vi "MeasLeakRate.vi"() -> ()   [LabVIEW 2011]
uses:
  <vilib>/Analysis/NI_AALPro.lvlib
panel:
  out "Pfit array":dbl[](array[numeric])=[-0.7941019304586632, -1.11]
  out "tFit array":dbl[](array[numeric])=[-20.0, 0.0]
  in  "tFit":dbl=10.0
  out "leak rate":dbl=-0.015794903477066843
  out "Polynomial Coefficients":dbl[](array[numeric])=[0.21180227710532212, -0.015794903477066843]
  out "Best Polynomial Fit":dbl[](array[numeric])=[0.21180227710532212, 0.22319040251225147, 0.23459432282271855, 0.24599824313318563, 0.257386368540115, 0.2688060837540049, 0.28019420916104915, 0.29158233456797844, 0.3029704599749078, 0.31435858538195205, 0.3257467107888814, 0.3371190412923879, 0.34849137179589446, 0.35987949720282375, 0.37128341751329086, 0.3826715429202202, 0.3940754632306873, 0.4054635886376166, 0.41685171404454596, 0.428255634355013, 0.43962796485851957, 0.45100029536202607, 0.4623884207689554, 0.47377654617588477, 0.48516467158292903, 0.49653700208643553, 0.5079409223967877, 0.5193132529002942, 0.5306855834038007, 0.5420737088107301, 0.5534776291211971, 0.5648657545282414, 0.5762538799351707, 0.5876735951490606, 0.59906172055599, 0.610465640866457, 0.6218379713699635, 0.6332260967768929, 0.6446142221839373, 0.6559865526873288, 0.667374678094373, 0.6787470085978795, 0.6901509289082317, 0.701539054315276, 0.7129271797222052, 0.7242837153221742, 0.7356718407292184, 0.7470757610396854, 0.7584480915430771, 0.7698520118535441, 0.7812401372604734, 0.7926124677639799, 0.8040005931710241, 0.8153729236744158, 0.8267610490814601, 0.8381333795849666, 0.8495215049918958, 0.8609096303988253, 0.8723135507092923, 0.8837016761162217]
  out "weight array":dbl[](array[numeric])=[1.0, 0.9304378473743352, 0.8656280206959002, 0.8053325349226013, 0.7493118702139018, 0.6970486998519578, 0.6485604918048629, 0.6034452278869568, 0.5614682788434552, 0.5224113367356974, 0.48607127959631125, 0.4523043432308019, 0.42088316568580814, 0.391605626676799, 0.3643282616568307, 0.3389848035136151, 0.3153727520215804, 0.2934347445114793, 0.2730227920280988, 0.254005337094879, 0.2363598138676975, 0.2199401093320528, 0.20464060187819116, 0.19040536109693249, 0.17716035430743396, 0.16485318319590794, 0.15337030310847227, 0.14271580554234622, 0.13280146637772186, 0.12356351050464263, 0.1149566704860605, 0.10696003702829307, 0.0995196666076842, 0.09257834684880129, 0.08613839775547324, 0.08013841114202638, 0.07457126750886783, 0.0693839296169267, 0.06455743411509868, 0.06007268699843237, 0.05589390157677298, 0.05201100230461187, 0.04838816596555581, 0.045022180979351074, 0.041890341154525154, 0.038984154900943556, 0.03627233316771518, 0.0337457768453816, 0.031401487957797174, 0.0292142112925875, 0.02718200786781411, 0.02529369813118136, 0.023534214041295513, 0.02189931327407275, 0.020375949901689627, 0.01896045091502129, 0.017641521134619163, 0.01641433894890389, 0.015270995021825278, 0.014208711735371296]
  out "dtArray":dbl[](array[numeric])=[0.0, -0.7209999999977299, -1.4429999999993015, -2.165000000000873, -2.885999999998603, -3.6089999999967404, -4.330000000001746, -5.050999999999476, -5.771999999997206, -6.493000000002212, -7.213999999999942, -7.934000000001106, -8.65400000000227, -9.375, -10.097000000001572, -10.817999999999302, -11.540000000000873, -12.260999999998603, -12.981999999996333, -13.703999999997905, -14.423999999999069, -15.144000000000233, -15.864999999997963, -16.585999999995693, -17.3070000000007, -18.027000000001863, -18.74899999999616, -19.468999999997322, -20.188999999998487, -20.909999999996217, -21.631999999997788, -22.353000000002794, -23.074000000000524, -23.79699999999866, -24.51799999999639, -25.239999999997963, -25.959999999999127, -26.680999999996857, -27.402000000001863, -28.12199999999575, -28.843000000000757, -29.56300000000192, -30.284999999996217, -31.006000000001222, -31.726999999998952, -32.445999999996275, -33.16700000000128, -33.88900000000285, -34.60899999999674, -35.33099999999831, -36.05199999999604, -36.771999999997206, -37.49300000000221, -38.2129999999961, -38.934000000001106, -39.65400000000227, -40.375, -41.09599999999773, -41.8179999999993, -42.53899999999703]
  out "t_array":dbl[](array[numeric])=[54993.193, 54992.472, 54991.75, 54991.028, 54990.307, 54989.584, 54988.863, 54988.142, 54987.421, 54986.7, 54985.979, 54985.259, 54984.539, 54983.818, 54983.096, 54982.375, 54981.653, 54980.932, 54980.211, 54979.489, 54978.769, 54978.049, 54977.328, 54976.607, 54975.886, 54975.166, 54974.444, 54973.724, 54973.004, 54972.283, 54971.561, 54970.84, 54970.119, 54969.396, 54968.675, 54967.953, 54967.233, 54966.512, 54965.791, 54965.071, 54964.35, 54963.63, 54962.908, 54962.187, 54961.466, 54960.747, 54960.026, 54959.304, 54958.584, 54957.862, 54957.141, 54956.421, 54955.7, 54954.98, 54954.259, 54953.539, 54952.818, 54952.097, 54951.375, 54950.654]
  out "P_array":dbl[](array[numeric])=[-1.11, -1.1, -1.1, -1.1, -1.1, -1.12, -1.11, -1.1, -0.99, -0.82, -0.36, 4.91, 7.07, 8.7, 7.720000000000001, 6.69, 4.43, 3.14, 1.85, 0.05, -0.49, -0.74, -1.12, -1.12, -1.12, -1.12, -1.12, -1.12, -1.12, -1.12, -1.12, -1.12, -1.12, -1.12, -1.12, -1.12, -1.12, -1.13, -1.13, -1.13, -1.12, -1.12, -1.13, -1.13, -1.13, -1.12, -1.12, -1.13, -1.12, -1.12, -1.12, -1.12, -1.14, -1.14, -1.14, -1.12, -1.12, -1.12, -1.13, -1.13]
  out "angle (°)":dbl
  out "Status":string
  out "error out":errorcluster
  out "T-T0,P":cluster{"element":dbl, "element":dbl}[](array[cluster])
  out "XY Graph":cluster{"Value":dbl[], "Value":dbl[]}[](graph)=[{"Value"=[0.0, -0.7209999999977299, -1.4429999999993015, -2.165000000000873, -2.885999999998603, -3.6089999999967404, -4.330000000001746, -5.050999999999476, -5.771999999997206, -6.493000000002212, -7.213999999999942, -7.934000000001106, -8.65400000000227, -9.375, -10.097000000001572, -10.817999999999302, -11.540000000000873, -12.260999999998603, -12.981999999996333, -13.703999999997905, -14.423999999999069, -15.144000000000233, -15.864999999997963, -16.585999999995693, -17.3070000000007, -18.027000000001863, -18.74899999999616, -19.468999999997322, -20.188999999998487, -20.909999999996217, -21.631999999997788, -22.353000000002794, -23.074000000000524, -23.79699999999866, -24.51799999999639, -25.239999999997963, -25.959999999999127, -26.680999999996857, -27.402000000001863, -28.12199999999575, -28.843000000000757, -29.56300000000192, -30.284999999996217, -31.006000000001222, -31.726999999998952, -32.445999999996275, -33.16700000000128, -33.88900000000285, -34.60899999999674, -35.33099999999831, -36.05199999999604, -36.771999999997206, -37.49300000000221, -38.2129999999961, -38.934000000001106, -39.65400000000227, -40.375, -41.09599999999773, -41.8179999999993, -42.53899999999703], "Value"=[-1.11, -1.1, -1.1, -1.1, -1.1, -1.12, -1.11, -1.1, -0.99, -0.82, -0.36, 4.91, 7.07, 8.7, 7.720000000000001, 6.69, 4.43, 3.14, 1.85, 0.05, -0.49, -0.74, -1.12, -1.12, -1.12, -1.12, -1.12, -1.12, -1.12, -1.12, -1.12, -1.12, -1.12, -1.12, -1.12, -1.12, -1.12, -1.13, -1.13, -1.13, -1.12, -1.12, -1.13, -1.13, -1.13, -1.12, -1.12, -1.13, -1.12, -1.12, -1.12, -1.12, -1.14, -1.14, -1.14, -1.12, -1.12, -1.12, -1.13, -1.13]}, {"Value"=[-20.0, 0.0], "Value"=[-0.7941019304586632, -1.11]}]
  out "T,P":cluster{"element":dbl, "element":dbl}[](array[cluster])
  in  "Control Valve Local":bool
  in  "Exhaust Close":bool
  in  "Exhaust Open":bool
  in  "Control Close":bool
  in  "Control Open":bool
  in  "reset":bool
  in  "# points to watch":i32=60
  out "leak rate (torr/min)":string="-0.948"
  out "P":dbl=-1.11
  out "first":bool
  in  "interval (s)":dbl=0.5
  in  "stop":bool
  out "P(torr)":string=" -1.11"
  # "Pressure control valve:"
  # "Exahaust valve:"
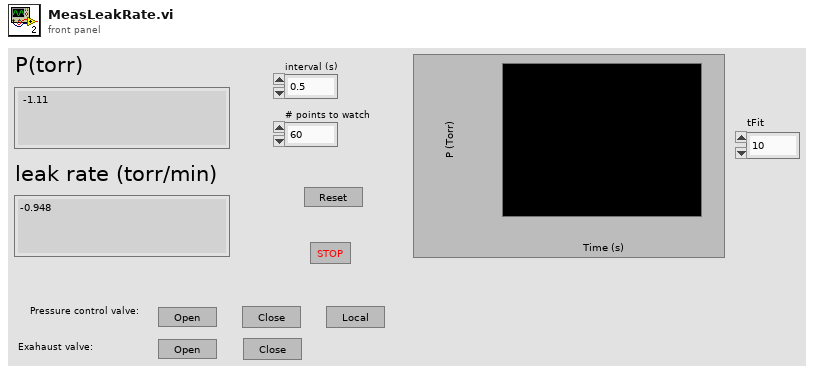
[diagram p1: front panel]
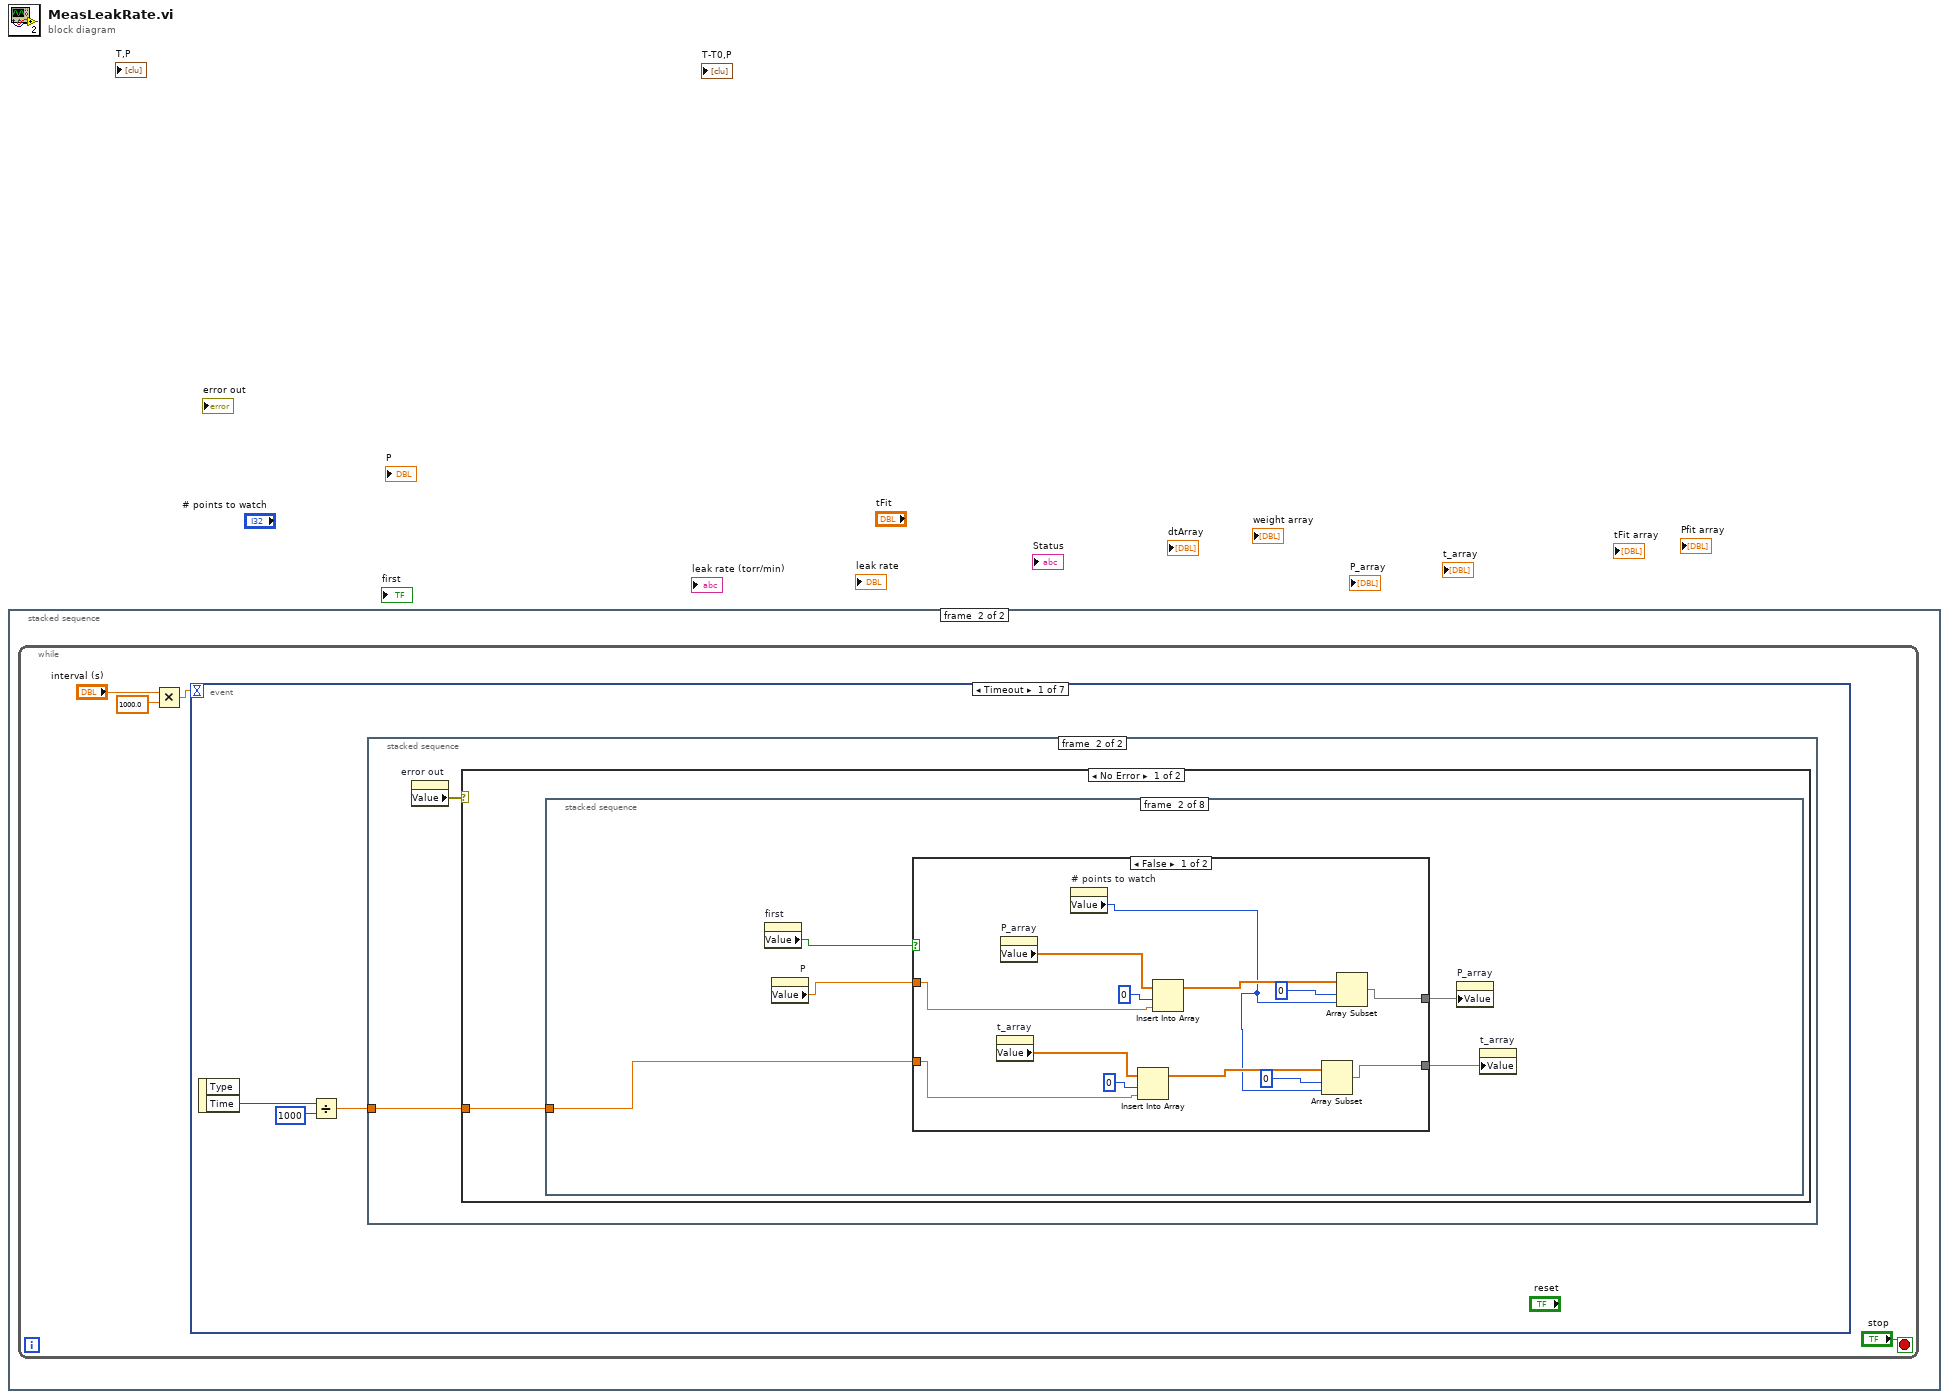
[diagram p0: block diagram]
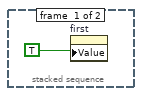
[diagram p2: hidden frame]
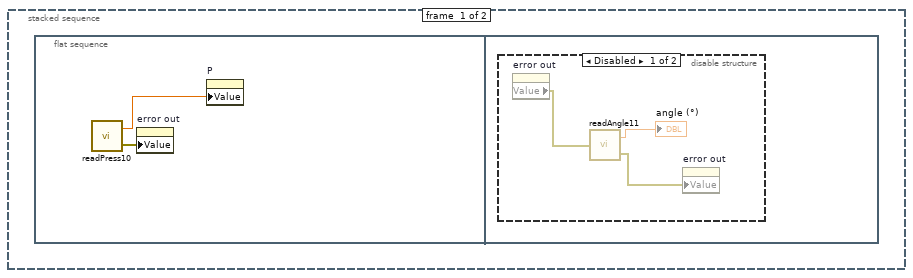
[diagram p3: hidden frame]
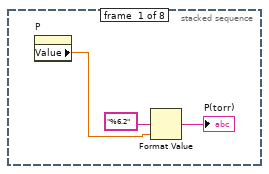
[diagram p5: hidden frame]
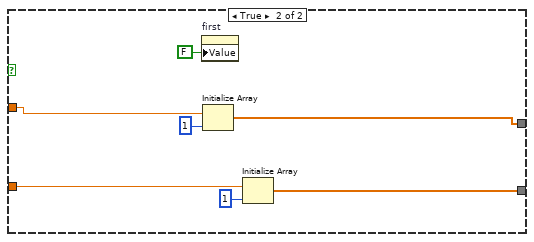
[diagram p6: hidden frame]
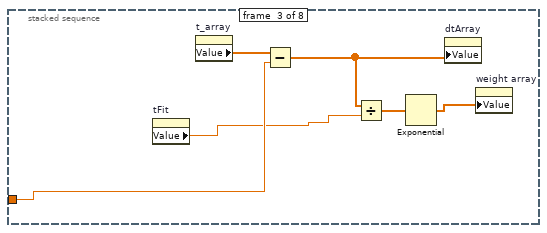
[diagram p7: hidden frame]
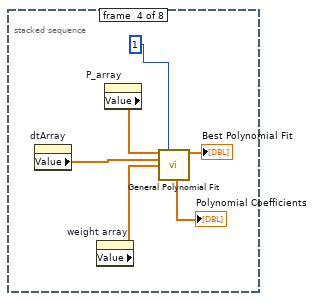
[diagram p8: hidden frame]
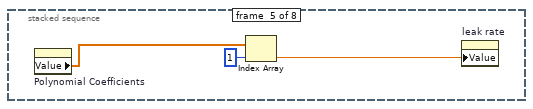
[diagram p9: hidden frame]
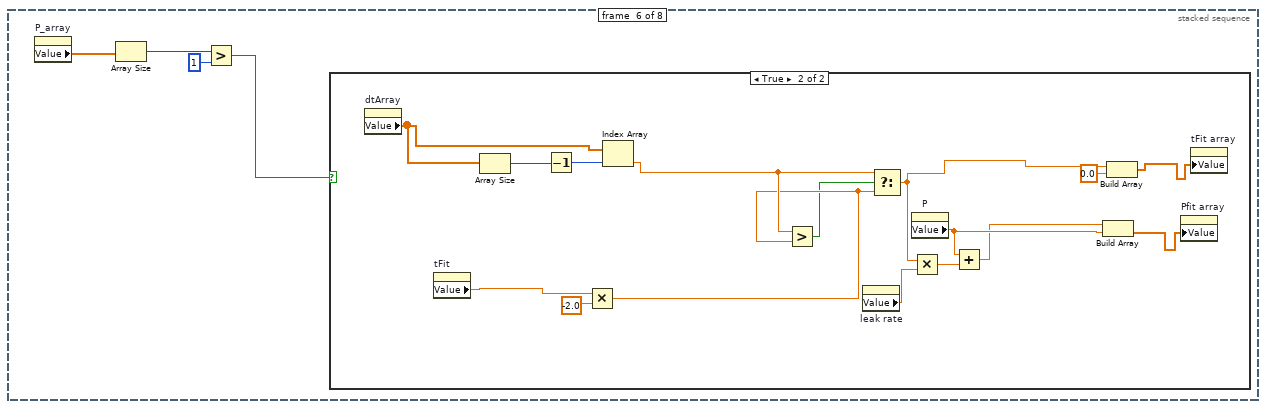
[diagram p10: hidden frame]
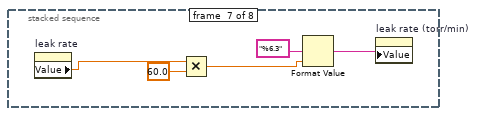
[diagram p12: hidden frame]
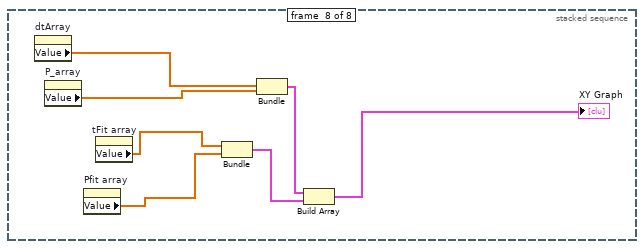
[diagram p13: hidden frame]
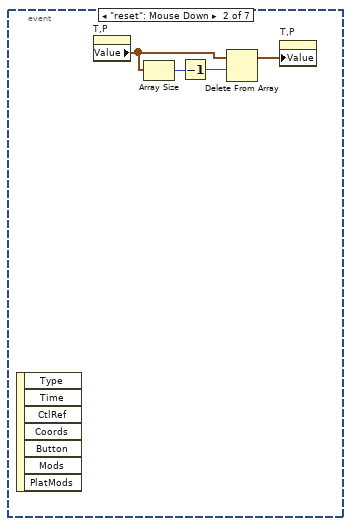
[diagram p15: hidden frame]
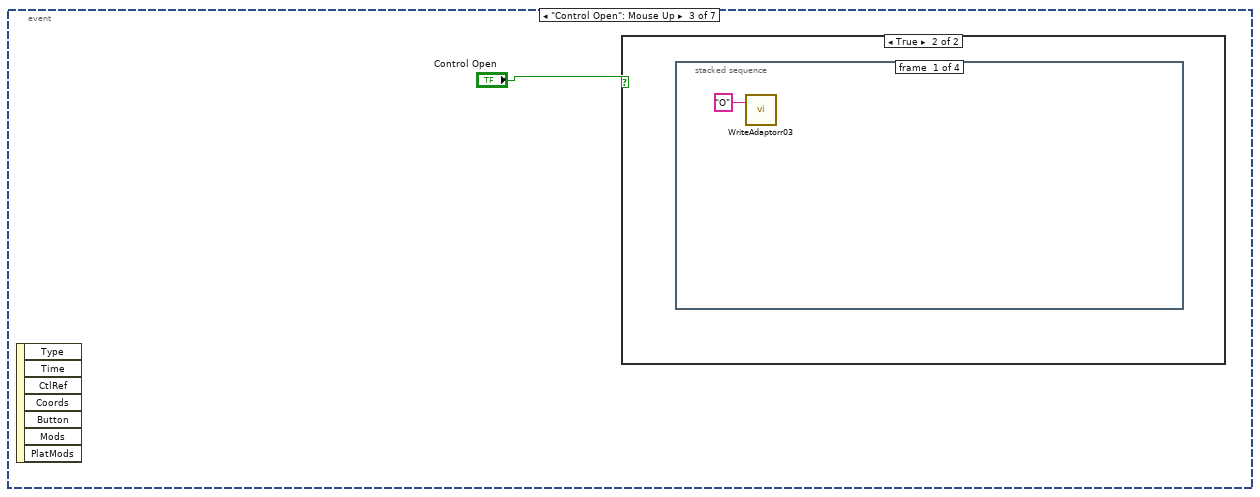
[diagram p16: hidden frame]
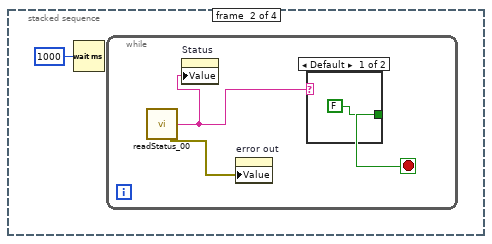
[diagram p18: hidden frame]
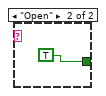
[diagram p19: hidden frame]
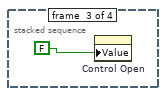
[diagram p20: hidden frame]
diagram:
  n1 = stacked-sequence {
    frame #0 {
      n2 = property on="first" class="Bool (strict)"("Value"=TRUE ("first")) -> ()  [unwired: 2 in, 2 out]
    }
    frame #1 {
      n3 = while {
        stop <- "stop" stop-if-true
        n4 = Multiply(x="interval (s)", y=1000.0) -> (x*y=w3:dbl)
        n5 = event shown="[0] Timeout" {
          selector: _ -> [_ _ _ _ _ _ _]
          dyn-events: _ -> [_ _ _ _ _ _ _]
          timeout: w3 -> [_ _ _ _ _ _ _]
          event Timeout {
            n6 = event-data() -> ("Time"=w8:u32)  [unwired: 1 in, 1 out]
            n7 = Divide(x=w8, y=u32 1000) -> (x/y=w6:dbl)
            n8 = stacked-sequence {
              tunnel: w6 -> [_ w14]
              frame #0 {
                n9 = flat-sequence {
                  frame #0 {
                    n10 = call "readPress10.vi"() -> ("P"=w10:dbl, "error out"=w9:errorcluster)  [unwired: 1 in]
                    n11 = property on="error out" class="Clust (strict)"("Value"=w9) -> ()  [unwired: 2 in, 2 out]
                    n12 = property on="P" class="DigNum (strict)"("Value"=w10) -> ()  [unwired: 2 in, 2 out]
                  }
                  frame #1 {
                    n13 = disable-structure shown="Disabled" {
                      frame Disabled {
                        n14 = property on="error out" class="Clust (strict)"() -> ("Value"=w12:errorcluster)  [unwired: 2 in, 2 out]
                        n15 = call "readAngle11.vi"("error in"=w12) -> ("angle"=→"angle (°)":dbl, "error out"=w11:errorcluster)
                        n16 = property on="error out" class="Clust (strict)"("Value"=w11) -> ()  [unwired: 2 in, 2 out]
                      }
                      frame Enabled {
                      }
                    }
                  }
                }
              }
              frame #1 {
                n17 = property on="error out" class="Clust (strict)"() -> ("Value"=w15:errorcluster)  [unwired: 2 in, 2 out]
                n18 = case shown="No Error" w15 {
                  tunnel: w14 -> [w16 _]
                  frame No Error {
                    n19 = stacked-sequence {
                      tunnel: w16 -> [_ w21 w48 _ _ _ _ _]
                      frame #0 {
                        n20 = property on="P" class="DigNum (strict)"() -> ("Value"=w17:dbl)  [unwired: 2 in, 2 out]
                        n21 = Format Value(format string="%6.2", value (0)=w17) -> (output string=→"P(torr)":string)  [unwired: 1 in]
                      }
                      frame #1 {
                        n22 = property on="first" class="Bool (strict)"() -> ("Value"=w24:bool)  [unwired: 2 in, 2 out]
                        n23 = property on="P" class="DigNum (strict)"() -> ("Value"=w23:dbl)  [unwired: 2 in, 2 out]
                        n24 = case shown="False" w24 {
                          tunnel: w23 -> [w34 w42]
                          tunnel: [w33 w41] -> w22
                          tunnel: w21 -> [w27 w39]
                          tunnel: [w28 w38] -> w20
                          frame False {
                            n25 = property on="t_array" class="Arr (strict)"() -> ("Value"=w26:dbl[])  [unwired: 2 in, 2 out]
                            n26 = property on="P_array" class="Arr (strict)"() -> ("Value"=w32:dbl[])  [unwired: 2 in, 2 out]
                            n27 = property on="# points to watch" class="DigNum (strict)"() -> ("Value"=w25:i32)  [unwired: 2 in, 2 out]
                            n28 = Insert Into Array(array=w26, index=0, new element=w27) -> (w30:dbl[])
                            n29 = Insert Into Array(array=w32, index=0, new element=w34) -> (w36:dbl[])
                            n30 = Array Subset(array=w30, index=0, length=w25) -> (w28:dbl[])
                            n31 = Array Subset(array=w36, index=0, length=w25) -> (w33:dbl[])
                          }
                          frame True {
                            n32 = property on="first" class="Bool (strict)"("Value"=FALSE ("first")) -> ()  [unwired: 2 in, 2 out]
                            n33 = Initialize Array(w42, 1 ("dimension size")) -> (w41:dbl[])
                            n34 = Initialize Array(w39, 1 ("dimension size")) -> (w38:dbl[])
                          }
                        }
                        n35 = property on="P_array" class="Arr (strict)"("Value"=w22) -> ()  [unwired: 2 in, 2 out]
                        n36 = property on="t_array" class="Arr (strict)"("Value"=w20) -> ()  [unwired: 2 in, 2 out]
                      }
                      frame #2 {
                        n37 = property on="tFit" class="DigNum (strict)"() -> ("Value"=w45:dbl)  [unwired: 2 in, 2 out]
                        n38 = property on="t_array" class="Arr (strict)"() -> ("Value"=w49:dbl[])  [unwired: 2 in, 2 out]
                        n39 = Subtract(x=w49, y=w48) -> (x-y=w47:dbl[])
                        n40 = Divide(x=w47, y=w45) -> (x/y=w50:dbl[])
                        n41 = Exponential(1:w50) -> (0:w46:dbl[])
                        n42 = property on="dtArray" class="Arr (strict)"("Value"=w47) -> ()  [unwired: 2 in, 2 out]
                        n43 = property on="weight array" class="Arr (strict)"("Value"=w46) -> ()  [unwired: 2 in, 2 out]
                      }
                      frame #3 {
                        n44 = property on="dtArray" class="Arr (strict)"() -> ("Value"=w55:dbl[])  [unwired: 2 in, 2 out]
                        n45 = property on="weight array" class="Arr (strict)"() -> ("Value"=w54:dbl[])  [unwired: 2 in, 2 out]
                        n46 = property on="P_array" class="Arr (strict)"() -> ("Value"=w56:dbl[])  [unwired: 2 in, 2 out]
                        n47 = call <vilib>:"General Polynomial Fit.vi"("Y"=w56, "polynomial order"=1, "X"=w55, "Weight"=w54) -> ("Best Polynomial Fit"=→"Best Polynomial Fit":dbl[], "Polynomial Coefficients"=→"Polynomial Coefficients":dbl[])  [unwired: 8 in, 2 out]
                      }
                      frame #4 {
                        n48 = property on="Polynomial Coefficients" class="Arr (strict)"() -> ("Value"=w59:dbl[])  [unwired: 2 in, 2 out]
                        n49 = Index Array(array=w59, index=1) -> (element=w57:dbl)
                        n50 = property on="leak rate" class="DigNum (strict)"("Value"=w57) -> ()  [unwired: 2 in, 2 out]
                      }
                      frame #5 {
                        n51 = property on="P_array" class="Arr (strict)"() -> ("Value"=w60:dbl[])  [unwired: 2 in, 2 out]
                        n52 = Array Size(array=w60) -> (size(s)=w61:i32)
                        n53 = Greater?(x=w61, y=1) -> (0:w63:bool)
                        n54 = case shown="True" w63 {
                          frame False {
                          }
                          frame True {
                            n55 = property on="dtArray" class="Arr (strict)"() -> ("Value"=w73:dbl[])  [unwired: 2 in, 2 out]
                            n56 = property on="tFit" class="DigNum (strict)"() -> ("Value"=w68:dbl)  [unwired: 2 in, 2 out]
                            n57 = Array Size(array=w73) -> (size(s)=w79:i32)
                            n58 = Decrement(x=w79) -> (x-1=w78:i32)
                            n59 = Multiply(x=w68, y=-2.0) -> (x*y=w67:dbl)
                            n60 = Index Array(array=w73, index=w78) -> (element=w74:dbl)
                            n61 = Greater?(x=w74, y=w67) -> (0:w66:bool)
                            n62 = property on="leak rate" class="DigNum (strict)"() -> ("Value"=w77:dbl)  [unwired: 2 in, 2 out]
                            n63 = Select(t=w74, s=w66, f=w67) -> (s? t:f=w70:dbl)
                            n64 = property on="P" class="DigNum (strict)"() -> ("Value"=w72:dbl)  [unwired: 2 in, 2 out]
                            n65 = Multiply(x=w70, y=w77) -> (x*y=w76:dbl)
                            n66 = Add(x=w72, y=w76) -> (x+y=w71:dbl)
                            n67 = Build Array(w71, w72) -> (w64:dbl[])
                            n68 = Build Array(w70, 0.0 ("element")) -> (w65:dbl[])
                            n69 = property on="Pfit array" class="Arr (strict)"("Value"=w64) -> ()  [unwired: 2 in, 2 out]
                            n70 = property on="tFit array" class="Arr (strict)"("Value"=w65) -> ()  [unwired: 2 in, 2 out]
                          }
                        }
                      }
                      frame #6 {
                        n71 = property on="leak rate" class="DigNum (strict)"() -> ("Value"=w82:dbl)  [unwired: 2 in, 2 out]
                        n72 = Multiply(x=w82, y=60.0) -> (x*y=w80:dbl)
                        n73 = Format Value(format string="%6.3", value (0)=w80) -> (output string=w84:string)  [unwired: 1 in]
                        n74 = property on="leak rate (torr/min)" class="Str"("Value"=w84) -> ()  [unwired: 2 in, 2 out]
                      }
                      frame #7 {
                        n75 = property on="dtArray" class="Arr (strict)"() -> ("Value"=w88:dbl[])  [unwired: 2 in, 2 out]
                        n76 = property on="P_array" class="Arr (strict)"() -> ("Value"=w89:dbl[])  [unwired: 2 in, 2 out]
                        n77 = property on="Pfit array" class="Arr (strict)"() -> ("Value"=w86:dbl[])  [unwired: 2 in, 2 out]
                        n78 = property on="tFit array" class="Arr (strict)"() -> ("Value"=w87:dbl[])  [unwired: 2 in, 2 out]
                        n79 = Bundle("Value"=w87, "Value"=w86) -> (w85:cluster{"Value":dbl[], "Value":dbl[]})  [unwired: 1 in]
                        n80 = Bundle("Value"=w88, "Value"=w89) -> (w91:cluster{"Value":dbl[], "Value":dbl[]})  [unwired: 1 in]
                        n81 = Build Array(w91, w85) -> (→"XY Graph":cluster{"Value":dbl[], "Value":dbl[]}[])
                      }
                    }
                  }
                  frame Error {
                  }
                }
              }
            }
          }
          event "reset": Mouse Down {
            n82 = event-data() -> ()  [unwired: 1 in, 7 out]
            n83 = property on="T,P" class="Arr (strict)"() -> ("Value"=w93:cluster{"element":dbl, "element":dbl}[])  [unwired: 2 in, 2 out]
            n84 = Array Size(array=w93) -> (size(s)=w95:i32)
            n85 = Decrement(x=w95) -> (x-1=w94:i32)
            n86 = Delete From Array(array=w93, length=w94) -> (array with subset deleted=w92:cluster{"element":dbl, "element":dbl}[])  [unwired: 1 in, 1 out]
            n87 = property on="T,P" class="Arr (strict)"("Value"=w92) -> ()  [unwired: 2 in, 2 out]
          }
          event "Control Open": Mouse Up {
            n88 = event-data() -> ()  [unwired: 1 in, 7 out]
            n89 = case shown="True" "Control Open" {
              frame False {
              }
              frame True {
                n90 = stacked-sequence {
                  frame #0 {
                    n91 = call "WriteAdaptorr03.vi"("string to write"="O") -> ()  [unwired: 1 in, 1 out]
                  }
                  frame #1 {
                    n92 = Wait (ms)(milliseconds to wait=u32 1000) -> ()  [unwired: 1 out]
                    n93 = while {
                      stop <- w100 stop-if-true
                      n94 = call "readStatus_00.vi"() -> ("Status"=w99:string, "error out"=w101:errorcluster)  [unwired: 1 in, 1 out]
                      n95 = property on="Status" class="Str"("Value"=w99) -> ()  [unwired: 2 in, 2 out]
                      n96 = property on="error out" class="Clust (strict)"("Value"=w101) -> ()  [unwired: 2 in, 2 out]
                      n97 = case shown="Default" w99 {
                        tunnel: [FALSE TRUE] -> w100
                        frame Default {
                        }
                        frame "Open" {
                        }
                      }
                    }
                  }
                  frame #2 {
                    n98 = property on="Control Open" class="Bool (strict)"("Value"=FALSE) -> ()  [unwired: 2 in, 2 out]
                  }
                  frame #3 {
                    n99 = call "WriteAdaptorr03.vi"("string to write"="D5") -> ()  [unwired: 1 in, 1 out]
                  }
                }
              }
            }
          }
          event "Control Close": Mouse Up {
            n100 = event-data() -> ()  [unwired: 1 in, 7 out]
            n101 = case shown="True" "Control Close" {
              frame False {
              }
              frame True {
                n102 = stacked-sequence {
                  frame #0 {
                    n103 = call "WriteAdaptorr03.vi"("string to write"="C") -> ()  [unwired: 1 in, 1 out]
                  }
                  frame #1 {
                    n104 = while {
                      stop <- w110 stop-if-true
                      n105 = call "readStatus_00.vi"() -> ("Status"=w108:string, "error out"=w109:errorcluster)  [unwired: 1 in, 1 out]
                      n106 = property on="Status" class="Str"("Value"=w108) -> ()  [unwired: 2 in, 2 out]
                      n107 = property on="error out" class="Clust (strict)"("Value"=w109) -> ()  [unwired: 2 in, 2 out]
                      n108 = case shown="\"Closed\"" w108 {
                        tunnel: [FALSE TRUE] -> w110
                        frame Default {
                        }
                        frame "Closed" {
                        }
                      }
                    }
                  }
                  frame #2 {
                    n109 = property on="Control Close" class="Bool (strict)"("Value"=FALSE) -> ()  [unwired: 2 in, 2 out]
                  }
                  frame #3 {
                    n110 = call "WriteAdaptorr03.vi"("string to write"="D5") -> ()  [unwired: 1 in, 1 out]
                  }
                }
              }
            }
          }
          event "Exhaust Open": Mouse Up {
            n111 = event-data() -> ()  [unwired: 1 in, 7 out]
            n112 = case shown="True" "Exhaust Open" {
              frame False {
              }
              frame True {
                n113 = call "set_vacuum.vi"("Remote"=TRUE ("Vac Remote"), "Atm"=FALSE ("Atm Exhaust"), "Vac Exhaust"=TRUE) -> ()
              }
            }
          }
          event "Exhaust Close": Mouse Up {
            n114 = event-data() -> ()  [unwired: 1 in, 7 out]
            n115 = case shown="True" "Exhaust Close" {
              frame False {
              }
              frame True {
                n116 = call "set_vacuum.vi"("Remote"=TRUE ("Vac Remote"), "Atm"=FALSE ("Atm Exhaust"), "Vac Exhaust"=FALSE) -> ()
              }
            }
          }
          event "Control Valve Local": Mouse Up {
            n117 = event-data() -> ()  [unwired: 1 in, 7 out]
            n118 = case shown="True" "Control Valve Local" {
              frame False {
              }
              frame True {
                n119 = call "WriteAdaptorr03.vi"("string to write"="D5") -> ()  [unwired: 1 in, 1 out]
              }
            }
          }
        }
      }
    }
  }
